vi "To Variant.vi"(0 "Obj in":refnum<class "SAM.lvclass">, 11 "error in (no error)":errorcluster) -> (4 "Obj out":refnum<class "SAM.lvclass">, 8 "Array":variant[](array[variant]), 15 "error out":errorcluster)   [LabVIEW 2020, in "SAM.lvclass"]
uses:
  SAM.lvclass
  SAM.lvclass/SAM.ctl
  AM/AM.lvclass
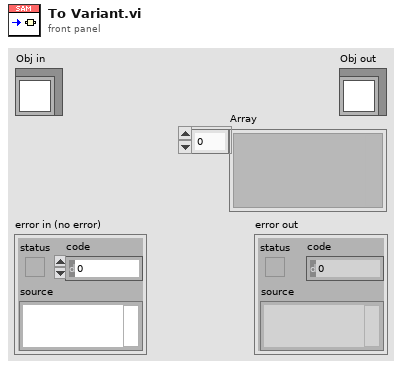
[diagram p1: front panel]
types:
  T1 = typedef "SAM.lvclass/Serialized.ctl" = cluster{"Frequency (Hz)":dbl, "Phase (0-1)":dbl}
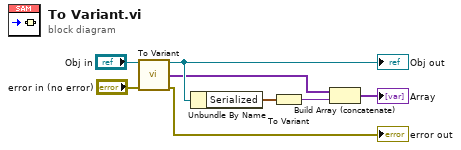
[diagram p0: block diagram]
diagram:
  n1 = call-parent "To Variant.vi"("Obj in"="Obj in", "error in (no error)"="error in (no error)") -> ("Obj out"=w3:refnum<class "SAM.lvclass">, "Array"=w2:variant[], "error out"=→"error out":errorcluster)  [unwired: 11 in]
  "Obj out" <- w3
  n2 = Unbundle By Name(w3) -> ("Serialized"=w4:T1)
  n3 = To Variant(anything=w4) -> (Variant=w5:variant)
  n4 = Build Array (concatenate)(w2, w5) -> (→"Array":variant[])
